vi "Test Glyph on Method Started Correct on Start Selective.vi"(8 "error in (no error)":errorcluster, 11 "Result Model Tests in":refnum<class "Result Model Test Enumeration.lvclass">) -> (0 "error out":errorcluster, 3 "Result Model Tests out":refnum<class "Result Model Test Enumeration.lvclass">)   [LabVIEW 2020, in "Result Model Test Enumeration.lvclass"]
uses:
  Result Model Test Enumeration.lvclass
  Result Model Test Enumeration.lvclass/Result Model Test Enumeration.ctl
  Result Model/Result Model.lvclass
  206db1ee-aa99-40b9-8881-171f2a77c34b.vi
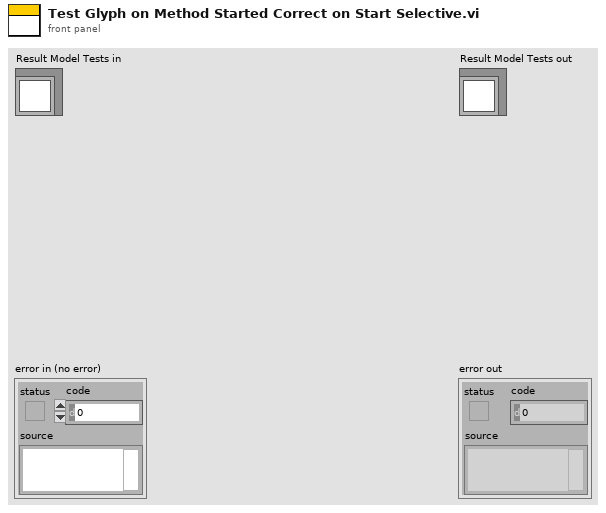
[diagram p1: front panel]
types:
  T1 = cluster{"Left Cell String":string, "Child Text":string[], "Child Tag":string, "Item Indent":i32, "Child Only?":bool, "Glyph Index":i32}[]
  T2 = cluster{"Left Cell String":string, "Child Text":string[], "Child Tag":string, "Item Indent":i32, "Child Only?":bool, "Glyph Index":i32}
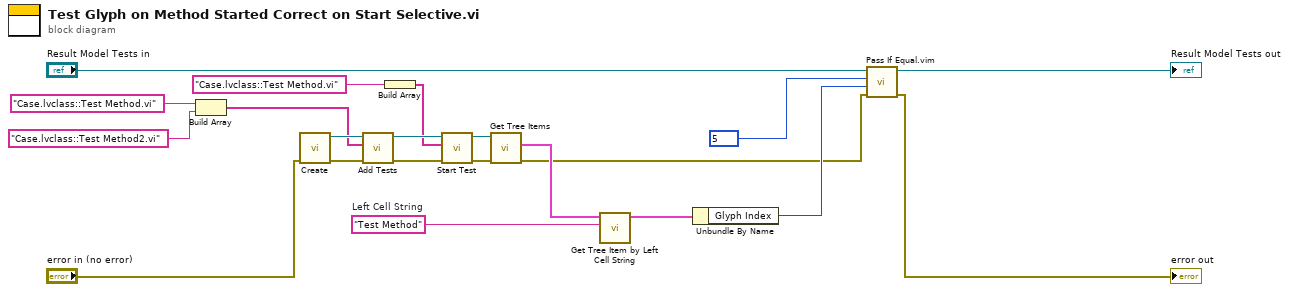
[diagram p0: block diagram]
diagram:
  w8 = "Test Method"  # Left Cell String
  n1 = Build Array("Case.lvclass::Test Method.vi" ("String"), "Case.lvclass::Test Method2.vi" ("String")) -> (w12:string[])
  n2 = call "Create.vi"("error in (no error)"="error in (no error)") -> ("error out"=w19:errorcluster, "Result Model out"=w20:refnum<class "Result Model.lvclass">)  [unwired: 9 in]
  n3 = call "Add Tests.vi"("error in (no error)"=w19, "Tests"=w12, "Result Model In"=w20) -> ("error out"=w18:errorcluster, "Result Model Out"=w5:refnum<class "Result Model.lvclass">)  [unwired: 7 in]
  n4 = Build Array("Case.lvclass::Test Method.vi" ("String")) -> (w1:string[])
  n5 = call "Start Test.vi"("error in (no error)"=w18, "Tests"=w1, "Result Model In"=w5) -> ("error out"=w6:errorcluster, "Result Model Out"=w4:refnum<class "Result Model.lvclass">)  [unwired: 7 in]
  n6 = call "Get Tree Items.vi"("error in (no error)"=w6, "Result Model In"=w4) -> ("error out"=w10:errorcluster, "Tree Items"=w16:T1)  [unwired: 7 in, 1 out]
  n7 = call "Get Tree Item by Left Cell String.vi"("Left Cell String"=w8, "Tree Items"=w16) -> ("Item"=w14:T2)  [unwired: 9 in]
  n8 = Unbundle By Name(w14) -> ("Glyph Index"=w13:i32)
  n9 = call "Pass If Equal.vim"("error in (no error)"=w10, "Actual"=w13, "Expected"=5 ("Listbox Symbol Ring Constant"), "LUnit Test Case In"="Result Model Tests in") -> ("error out"=→"error out":errorcluster, "LUnit Test Case Out"=→"Result Model Tests out":refnum<class "Result Model Test Enumeration.lvclass">)  [unwired: 6 in]
